vi "Flight Controller.vi"(8 "error IO":errorcluster) -> ()   [LabVIEW 2014]
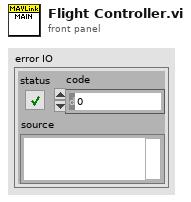
[diagram p1: front panel]
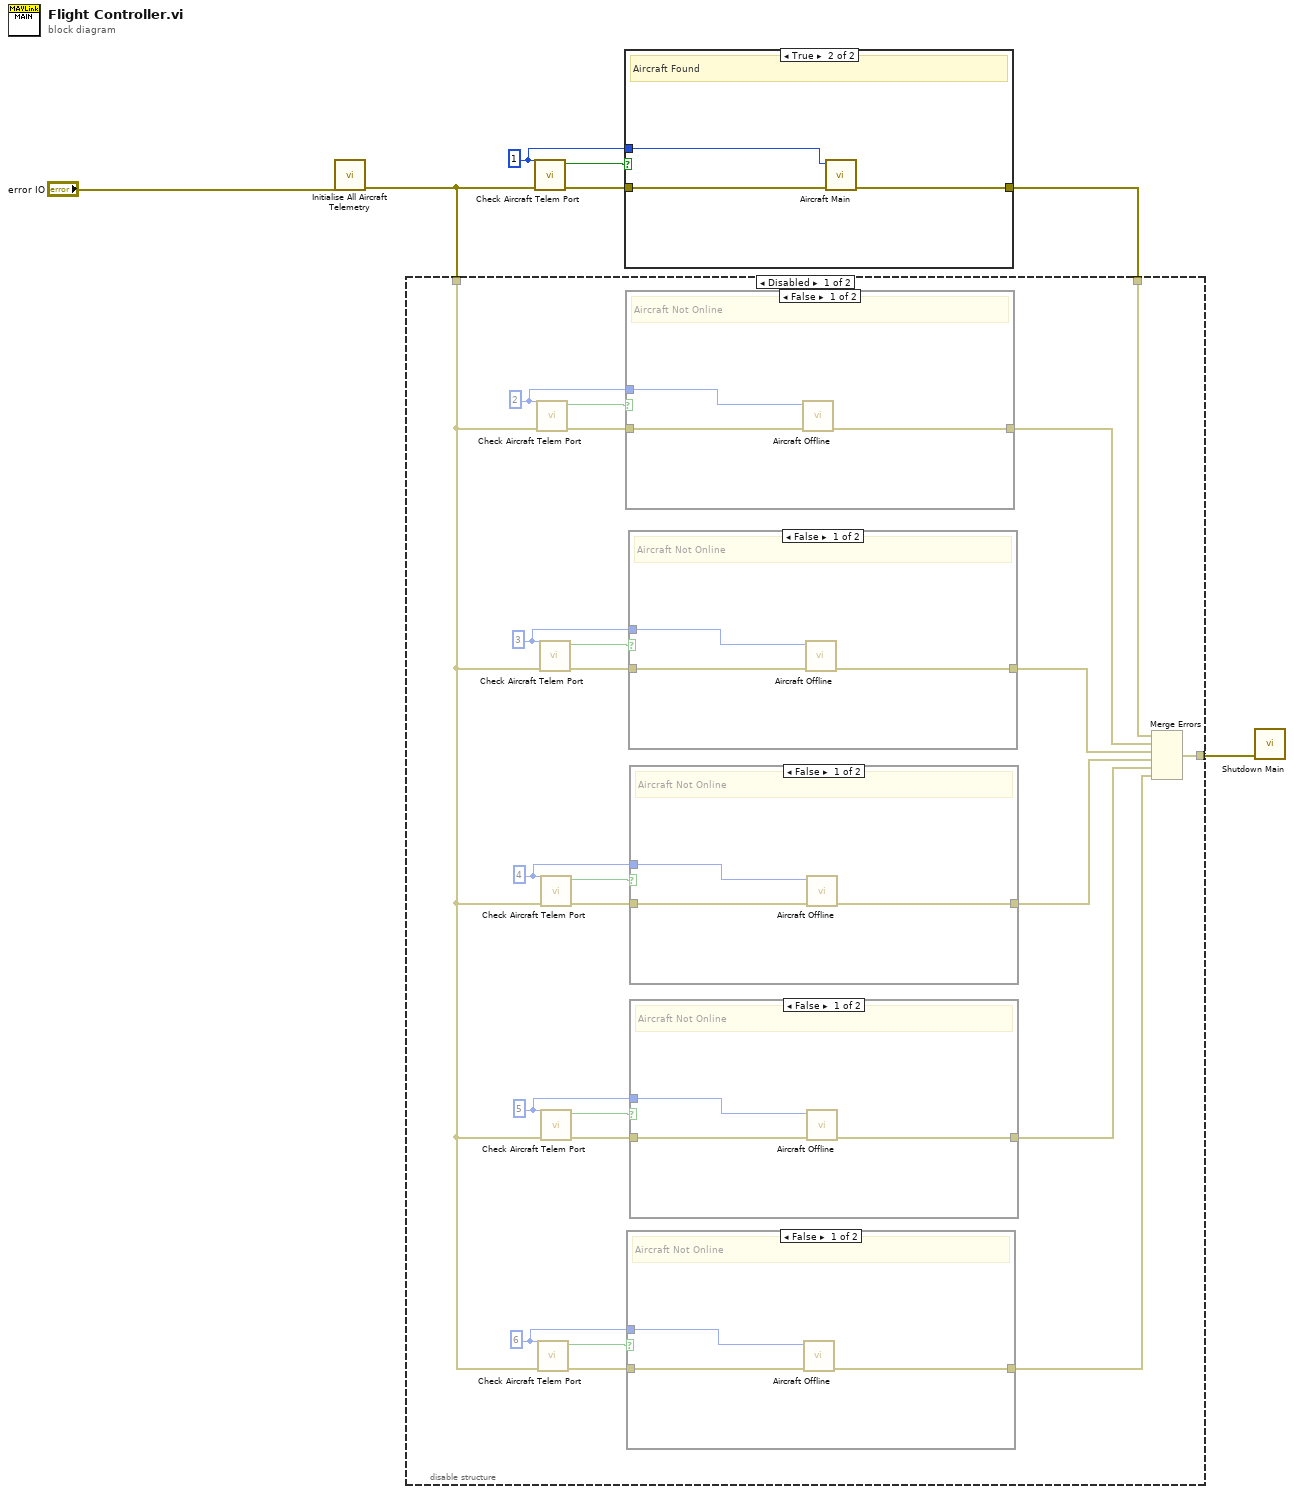
[diagram p0: block diagram]
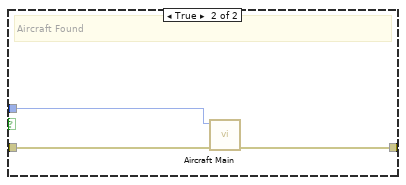
[diagram p2: hidden frame]
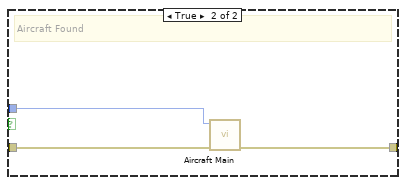
[diagram p3: hidden frame]
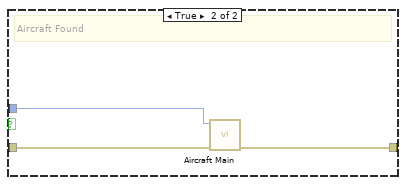
[diagram p4: hidden frame]
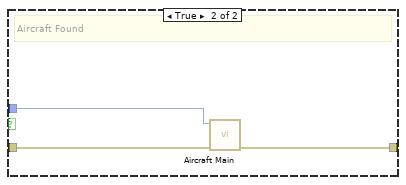
[diagram p5: hidden frame]
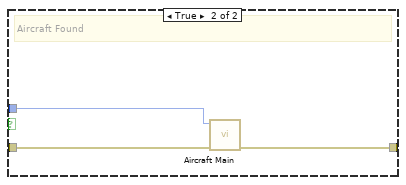
[diagram p6: hidden frame]
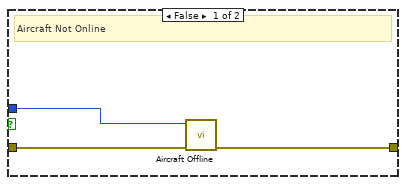
[diagram p8: hidden frame]
diagram:
  w5 = u8 1 ("Aircraft ID")
  n1 = call "Initialise All Aircraft Telemetry.vi"("error IO"="error IO") -> ("error out"=w4:errorcluster)  [unwired: 10 in]
  n2 = call "Check Aircraft Telem Port.vi"("Error In"=w4, "Aircraft ID"=w5) -> ("Error Out"=w6:errorcluster, "Telem Port Found"=w7:bool)  [unwired: 8 in]
  n3 = case shown="True" w7 {
    tunnel: w6 -> [w9 w13]
    tunnel: w5 -> [w10 w12]
    tunnel: [w8 w11] -> w3
    frame False {
      # "Aircraft Not Online"
      n4 = call "Aircraft Offline.vi"("Error In"=w9, "Aircraft ID"=w10) -> ("Error Out"=w8:errorcluster)  [unwired: 9 in]
    }
    frame True {
      # "Aircraft Found"
      n5 = call "Aircraft Main.vi"("error out"=w13, "Aircraft Index"=w12) -> ("error out 2"=w11:errorcluster)  [unwired: 9 in]
    }
  }
  n6 = disable-structure shown="Disabled" {
    disable-tunnel: w4 -> [w22 _]
    disable-tunnel: w3 -> [w21 w67]
    disable-tunnel: [w15 w67] -> w2
    frame Disabled {
      w25 = u8 6 ("Aircraft ID")
      w26 = u8 5 ("Aircraft ID")
      w31 = u8 4 ("Aircraft ID")
      w32 = u8 3 ("Aircraft ID")
      w14 = u8 2 ("Aircraft ID")
      n7 = call "Check Aircraft Telem Port.vi"("Error In"=w22, "Aircraft ID"=w14) -> ("Error Out"=w36:errorcluster, "Telem Port Found"=w35:bool)  [unwired: 8 in]
      n8 = call "Check Aircraft Telem Port.vi"("Error In"=w22, "Aircraft ID"=w25) -> ("Error Out"=w24:errorcluster, "Telem Port Found"=w23:bool)  [unwired: 8 in]
      n9 = call "Check Aircraft Telem Port.vi"("Error In"=w22, "Aircraft ID"=w32) -> ("Error Out"=w33:errorcluster, "Telem Port Found"=w34:bool)  [unwired: 8 in]
      n10 = call "Check Aircraft Telem Port.vi"("Error In"=w22, "Aircraft ID"=w31) -> ("Error Out"=w30:errorcluster, "Telem Port Found"=w29:bool)  [unwired: 8 in]
      n11 = call "Check Aircraft Telem Port.vi"("Error In"=w22, "Aircraft ID"=w26) -> ("Error Out"=w27:errorcluster, "Telem Port Found"=w28:bool)  [unwired: 8 in]
      n12 = case shown="False" w35 {
        tunnel: w36 -> [w62 w66]
        tunnel: w14 -> [w63 w65]
        tunnel: [w61 w64] -> w20
        frame False {
          # "Aircraft Not Online"
          n13 = call "Aircraft Offline.vi"("Error In"=w62, "Aircraft ID"=w63) -> ("Error Out"=w61:errorcluster)  [unwired: 9 in]
        }
        frame True {
          # "Aircraft Found"
          n14 = call "Aircraft Main.vi"("error out"=w66, "Aircraft Index"=w65) -> ("error out 2"=w64:errorcluster)  [unwired: 9 in]
        }
      }
      n15 = case shown="False" w23 {
        tunnel: w24 -> [w38 w42]
        tunnel: w25 -> [w39 w41]
        tunnel: [w37 w40] -> w16
        frame False {
          # "Aircraft Not Online"
          n16 = call "Aircraft Offline.vi"("Error In"=w38, "Aircraft ID"=w39) -> ("Error Out"=w37:errorcluster)  [unwired: 9 in]
        }
        frame True {
          # "Aircraft Found"
          n17 = call "Aircraft Main.vi"("error out"=w42, "Aircraft Index"=w41) -> ("error out 2"=w40:errorcluster)  [unwired: 9 in]
        }
      }
      n18 = case shown="False" w34 {
        tunnel: w33 -> [w56 w60]
        tunnel: w32 -> [w57 w59]
        tunnel: [w55 w58] -> w19
        frame False {
          # "Aircraft Not Online"
          n19 = call "Aircraft Offline.vi"("Error In"=w56, "Aircraft ID"=w57) -> ("Error Out"=w55:errorcluster)  [unwired: 9 in]
        }
        frame True {
          # "Aircraft Found"
          n20 = call "Aircraft Main.vi"("error out"=w60, "Aircraft Index"=w59) -> ("error out 2"=w58:errorcluster)  [unwired: 9 in]
        }
      }
      n21 = case shown="False" w29 {
        tunnel: w30 -> [w50 w54]
        tunnel: w31 -> [w51 w53]
        tunnel: [w49 w52] -> w18
        frame False {
          # "Aircraft Not Online"
          n22 = call "Aircraft Offline.vi"("Error In"=w50, "Aircraft ID"=w51) -> ("Error Out"=w49:errorcluster)  [unwired: 9 in]
        }
        frame True {
          # "Aircraft Found"
          n23 = call "Aircraft Main.vi"("error out"=w54, "Aircraft Index"=w53) -> ("error out 2"=w52:errorcluster)  [unwired: 9 in]
        }
      }
      n24 = case shown="False" w28 {
        tunnel: w27 -> [w44 w48]
        tunnel: w26 -> [w45 w47]
        tunnel: [w43 w46] -> w17
        frame False {
          # "Aircraft Not Online"
          n25 = call "Aircraft Offline.vi"("Error In"=w44, "Aircraft ID"=w45) -> ("Error Out"=w43:errorcluster)  [unwired: 9 in]
        }
        frame True {
          # "Aircraft Found"
          n26 = call "Aircraft Main.vi"("error out"=w48, "Aircraft Index"=w47) -> ("error out 2"=w46:errorcluster)  [unwired: 9 in]
        }
      }
      n27 = Merge Errors(w21, w20, w19, w18, w17, w16) -> (w15:errorcluster)
    }
    frame Enabled {
    }
  }
  n28 = call "Shutdown Main.vi"("error out"=w2) -> ()  [unwired: 11 in]
